vi "Make Versioned Name.vi"() -> (3 "versioned name":string)   [LabVIEW 2019, in "LMH-LINX.lvlib"]
uses:
  <vilib>/MakerHub/LINX/LMH-LINX.lvlib
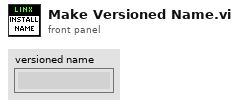
[diagram p1: front panel]
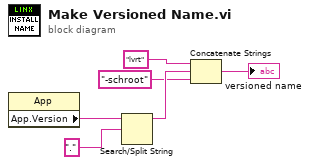
[diagram p0: block diagram]
diagram:
  n1 = property class="App"() -> ("App.Version"=w6:string)  [unwired: 2 in, 2 out]
  n2 = Search/Split String(string=w6, search string/char (-)=".") -> (substring before match=w4:string)  [unwired: 1 in, 2 out]
  n3 = Concatenate Strings("lvrt" ("search string/char (-)"), w4, "-schroot" ("search string/char (-)")) -> (→"versioned name":string)
